vi "demo-geometry.vi"() -> ()   [LabVIEW 2019]
uses:
  <vilib>/Rock Robotics/WPI/ThirdParty/JAS_Junk/TrajLib/Trajectory_Library.lvlib
  ROBOT_PICTURE.ctl
  <vilib>/Rock Robotics/WPI/ThirdParty/JAS_Junk/TrajLib/TRANSLATION2D.ctl
  <vilib>/Rock Robotics/WPI/ThirdParty/JAS_Junk/TrajLib/ROTATION2D.ctl
  <vilib>/Rock Robotics/WPI/ThirdParty/JAS_Junk/TrajLib/POSE2D.ctl
panel:
  out "Ball Angle From Robot":T1 {"SIN" format="%13.4f"; "COS" format="%13.4f"; "VALUE" format="%13.4f"}
  out "Ball Location From Robot":T2 {"Y" format="%14.3f"; "X" format="%14.3f"}
  out "Ball Location":T2 {"Y" format="%14.3f"; "X" format="%14.3f"}
  out "Robot POSE":T3 {"ROTATION"."SIN" format="%13.4f"; "ROTATION"."COS" format="%13.4f"; "ROTATION"."VALUE" format="%13.4f"; "TRANSLATION"."Y" format="%14.3f"; "TRANSLATION"."X" format="%14.3f"}
  out "BALL":bool=TRUE
  in  "Y  INCHES - BALL":dbl
  in  "X INCHES - BALL":dbl
  in  "ORIENTATION - DEG":dbl
  in  "Y  INCHES":dbl
  in  "X INCHES":dbl
  out "2D Picture":T4
  # "ROBOT"
  # "BALL"
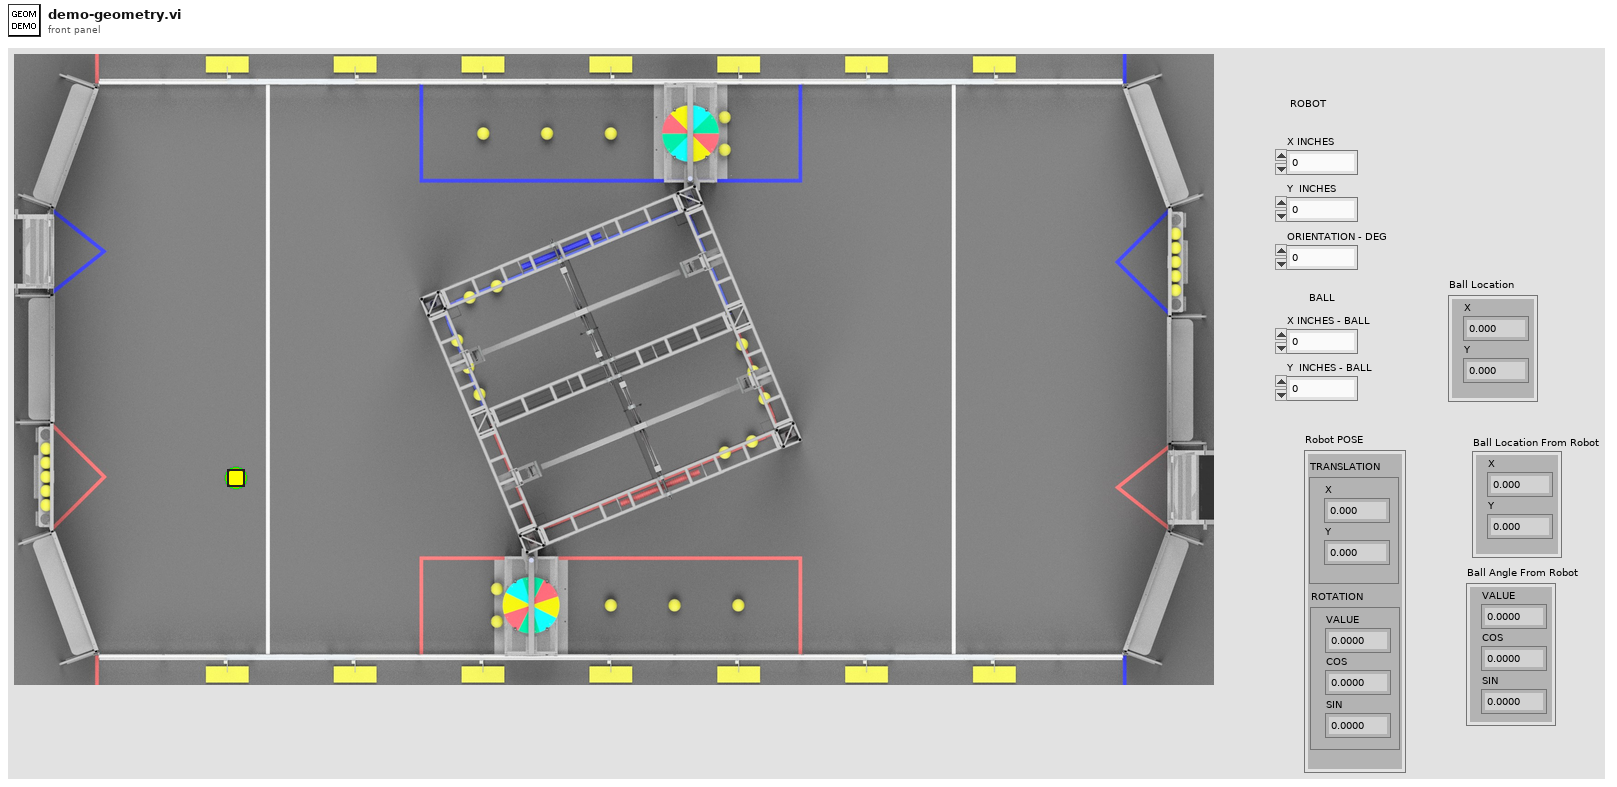
[diagram p1: front panel]
types:
  T1 = typedef "Trajectory_Library.lvlib/ROTATION2D.ctl" = cluster{"VALUE":dbl, "COS":dbl, "SIN":dbl}
  T2 = typedef "Trajectory_Library.lvlib/TRANSLATION2D.ctl" = cluster{"X":dbl, "Y":dbl}
  T3 = typedef "Trajectory_Library.lvlib/POSE2D.ctl" = cluster{"TRANSLATION":T2, "ROTATION":T1}
  T4 = typedef "ROBOT_PICTURE.ctl" = picture
  T5 = typedef "Rotated_Picture_TypeDef.ctl" = cluster{"ONE-8-bit pixmap":u8[][], "Two-Array":cdb[][], "Three-Numeric":i32, "Four-Numeric":i32, "Five-Numeric":cdb, "Six-colors":u32[], "Seven-new element/subarray":u32, "Eight-Cluster":cluster{"[0]":i32, "[1]":i32}}
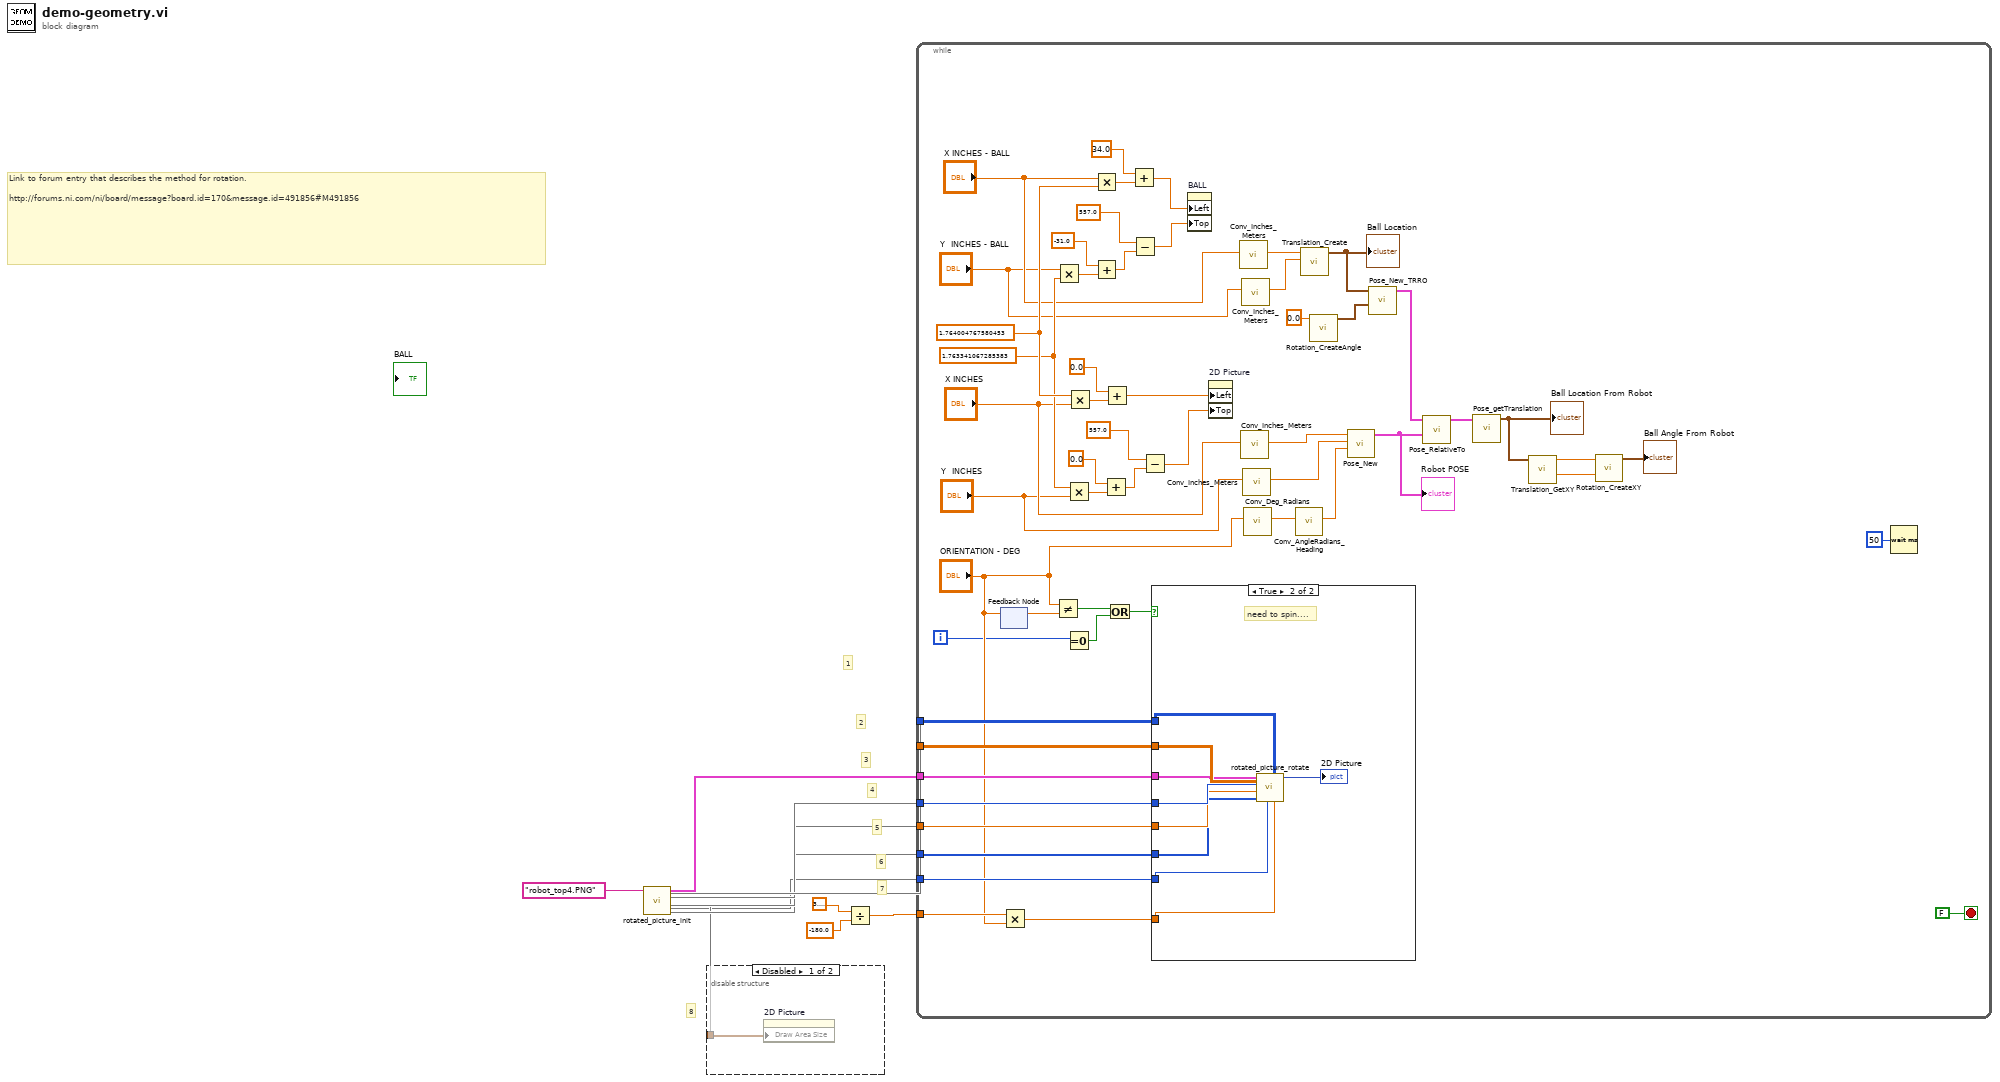
[diagram p0: block diagram]
diagram:
  # "8"
  # "7"
  # "6"
  # "5"
  # "4"
  # "3"
  # "2"
  # "1"
  # "Link to forum entry that describes the method for rotation.\n\nhttp://forums.ni.com/ni/board/message?board.id=170&message.id=491856#M491856"
  n1 = call "rotated_picture_init.vi"("Picture FIle Name"="robot_top4.PNG" ("name or relative path")) -> (0:w3, 1:w4, 2:w5, "RotatedPictureInfo"=w6:T5, 4:w1, 5:w7, 6:w2, 7:w8)  [unwired: 3 in]
  n2 = disable-structure shown="Disabled" {
    disable-tunnel: w2 -> [w13 _]
    frame Disabled {
      n3 = property on="2D Picture" class="Pict (strict)"("Draw Area Size"=w13) -> ()  [unwired: 2 in, 2 out]
    }
    frame Enabled {
    }
  }
  n4 = Divide(x=3.141592653589793, y=-180.0 ("value")) -> (x/y=w10:dbl)
  n5 = while {
    tunnel: w8 -> [w68]
    tunnel: w7 -> [w67]
    tunnel: w4 -> [w66]
    tunnel: w3 -> [w65]
    tunnel: w10 -> [w64]
    tunnel: w6 -> [w63]
    tunnel: w5 -> [w62]
    tunnel: w1 -> [w58]
    i -> [w14]
    stop <- FALSE stop-if-true
    w39 = 1.763341067285383
    w46 = 1.764004767580453
    n6 = feedback-in #1("ORIENTATION - DEG") -> ()
    n7 = feedback #1() -> (w57:dbl)  [unwired: 1 in]
    n8 = Multiply(x=w64, y="ORIENTATION - DEG") -> (x*y=w60:dbl)
    n9 = Not Equal?(x="ORIENTATION - DEG", y=w57) -> (x != y?=w16:bool)
    n10 = Multiply(x="Y  INCHES - BALL", y=w39) -> (x*y=w44:dbl)
    n11 = Multiply(x=w39, y="Y  INCHES") -> (x*y=w54:dbl)
    n12 = Equal To 0?(x=w14) -> (x = 0?=w15:bool)
    n13 = Multiply(x=w46, y="X INCHES") -> (x*y=w56:dbl)
    n14 = Multiply(x="X INCHES - BALL", y=w46) -> (x*y=w48:dbl)
    n15 = Add(x=-31.0, y=w44) -> (x+y=w41:dbl)
    n16 = Add(x=0.0, y=w54) -> (x+y=w50:dbl)
    n17 = Add(x=0.0, y=w56) -> (x+y=w51:dbl)
    n18 = Or(x=w16, y=w15) -> (x .or. y?=w17:bool)
    n19 = Add(x=34.0, y=w48) -> (x+y=w45:dbl)
    n20 = Subtract(x=557.0, y=w41) -> (x-y=w40:dbl)
    n21 = Subtract(x=557.0, y=w50) -> (x-y=w49:dbl)
    n22 = case shown="True" w17 {
      tunnel: w68 -> [_ w76]
      tunnel: w67 -> [_ w75]
      tunnel: w66 -> [_ w72]
      tunnel: w65 -> [_ w71]
      tunnel: w63 -> [_ w74]
      tunnel: w62 -> [_ w73]
      tunnel: w60 -> [_ w69]
      tunnel: w58 -> [_ w70]
      frame False {
        # "Leave as is..."
      }
      frame True {
        # "need to spin...."
        n23 = call "rotated_picture_rotate.vi"(4:w69, 5:w76, 6:w70, 7:w75, 8:w71, "Angle"=w72, 10:w73, "RotatedPictureInfo"=w74) -> ("new picture"=→"2D Picture":picture)  [unwired: 3 in]
      }
    }
    n24 = property on="BALL" class="Bool (strict)"("Left"=w45, "Top"=w40) -> ()  [unwired: 2 in, 2 out]
    n25 = property on="2D Picture" class="Pict (strict)"("Left"=w51, "Top"=w49) -> ()  [unwired: 2 in, 2 out]
    n26 = call <vilib>:"Conv_Inches_Meters.vi"("INCH"="X INCHES - BALL") -> ("Meters"=w30:dbl)  [unwired: 10 in]
    n27 = call <vilib>:"Conv_Inches_Meters.vi"("INCH"="X INCHES") -> ("Meters"=w34:dbl)  [unwired: 10 in]
    n28 = call <vilib>:"Conv_Inches_Meters.vi"("INCH"="Y  INCHES - BALL") -> ("Meters"=w29:dbl)  [unwired: 10 in]
    n29 = call <vilib>:"Conv_Inches_Meters.vi"("INCH"="Y  INCHES") -> ("Meters"=w33:dbl)  [unwired: 10 in]
    n30 = call <vilib>:"Conv_Deg_Radians.vi"("Degress"="ORIENTATION - DEG") -> ("Radians"=w35:dbl)  [unwired: 10 in]
    n31 = call <vilib>:"Conv_AngleRadians_Heading.vi"("Radians"=w35) -> ("Heading"=w26:dbl)  [unwired: 10 in]
    n32 = call <vilib>:"Translation_Create.vi"("Y"=w29, "X"=w30) -> ("TRANSLATION"=w28:T2)  [unwired: 9 in]
    "Ball Location" <- w28
    n33 = call <vilib>:"Rotation_CreateAngle.vi"("Angle"=0.0) -> ("ROTATION"=w23:T1)  [unwired: 10 in]
    n34 = call <vilib>:"Pose_New.vi"("Heading"=w26, "Y"=w33, "X"=w34) -> ("out POSe"=w25:T3)  [unwired: 8 in]
    "Robot POSE" <- w25
    n35 = call <vilib>:"Pose_New_TRRO.vi"("ROTATION"=w23, "TRANSLATION"=w28) -> ("outPOSE"=w27:T3)  [unwired: 9 in]
    n36 = call <vilib>:"Pose_RelativeTo.vi"("other POSE"=w25, "in POSE"=w27) -> ("out POSE"=w22:T3)  [unwired: 9 in]
    n37 = call <vilib>:"Pose_getTranslation.vi"("in POSE"=w22) -> ("outTRANSLATION"=w21:T2)  [unwired: 10 in]
    "Ball Location From Robot" <- w21
    n38 = call <vilib>:"Translation_GetXY.vi"("In Translation"=w21) -> ("Y"=w19:dbl, "X"=w20:dbl)  [unwired: 9 in]
    n39 = call <vilib>:"Rotation_CreateXY.vi"("Y or sine"=w19, "X or  cosine"=w20) -> ("ROTATION"=→"Ball Angle From Robot":T1)  [unwired: 9 in]
    n40 = Wait (ms)(milliseconds to wait=u32 50) -> ()  [unwired: 1 out]
  }
